vi "I32 to String.vi"(11 "Numeric":i32) -> (3 "String":string)   [LabVIEW 2014, in "SLL String.lvlib"]
uses:
  SLL String.lvlib
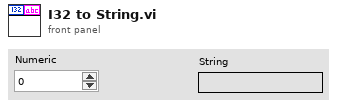
[diagram p1: front panel]
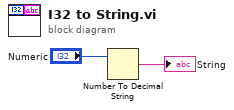
[diagram p0: block diagram]
diagram:
  n1 = Number To Decimal String(number="Numeric") -> (decimal integer string=→"String":string)  [unwired: 1 in]
